vi "create queue.vi"(8 "error in (no error)":errorcluster, 11 "name (unnamed)":string) -> (0 "error out":errorcluster, 3 "queue out":refnum<queue>)   [LabVIEW 2024, in "Ev Queued SM API.lvlib"]
doc: "The type of data that the queue will host is defined. The data type is a cluster containing a string for the status and a variant for the data."
uses:
  Ev Queued SM API.lvlib
  controls/State & Data Cluster.ctl
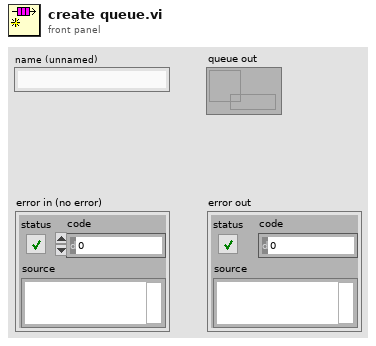
[diagram p1: front panel]
types:
  T1 = typedef "Ev Queued SM API.lvlib/State & Data Cluster.ctl" = cluster{"State":string, "Data":variant}
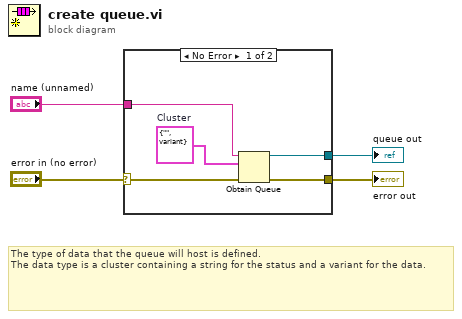
[diagram p0: block diagram]
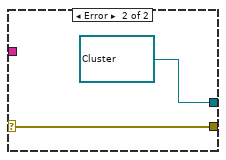
[diagram p2: hidden frame]
diagram:
  # "The type of data that the queue will host is defined. \nThe data type is a cluster containing a string for the status and a variant for the data."
  n1 = case shown="No Error" "error in (no error)" {
    selector: "error in (no error)" -> [w6 w11]
    tunnel: [w9 w11] -> w4
    tunnel: [w8 refnum<queue> refnum ("queue out")] -> w3
    tunnel: "name (unnamed)" -> [w5 _]
    frame No Error {
      w7 = T1 {"State"="", "Data"=variant}  # Cluster
      n2 = Obtain Queue(name (unnamed)=w5, element data type=w7, error in (no error)=w6) -> (queue out=w8:refnum<queue>, error out=w9:errorcluster)  [unwired: 2 in, 1 out]
    }
    frame Error {
    }
  }
  "error out" <- w4
  "queue out" <- w3
